vi "DestroyPublicEvents.vi"(8 "error in (no error)":errorcluster, 11 "SMO.Configurable":refnum<class "SMO.Configurable.lvclass">) -> (0 "error out":errorcluster, 3 "SMO.Configurable out":refnum<class "SMO.Configurable.lvclass">)   [LabVIEW 2013, in "SMO.Configurable.lvclass"]
uses:
  SMO.Configurable.lvclass
  src/SMO/SMO.lvclass
  SMO.Configurable.lvclass/SMO.Configurable.ctl
panel:
  # "For instructions on how to use the JKI State Machine Objects, examples and video tutorials, visit:\nhttp://jki.net/state-machine-objects/\n\nJKI State Machine Objects™\nhttp://jki.net/state-machine-objects/\nCopyright (C) 2005-2015, JKI <info@jki.net>\nALL RIGHTS RESERVED"
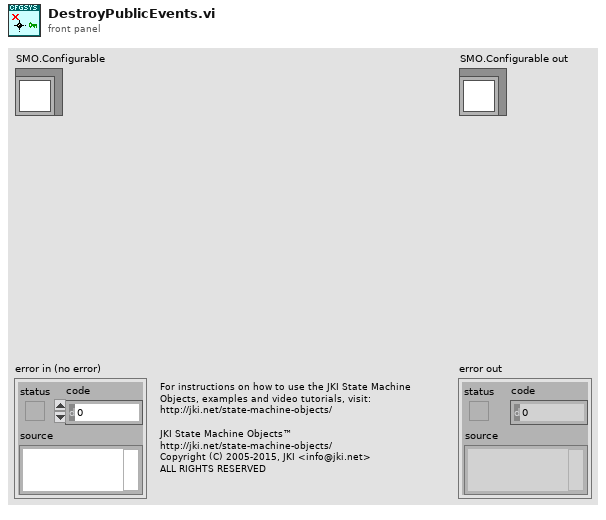
[diagram p1: front panel]
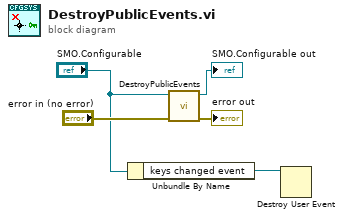
[diagram p0: block diagram]
diagram:
  n1 = Unbundle By Name("SMO.Configurable") -> ("keys changed event"=w1:refnum<user-event>)
  n2 = call-parent "DestroyPublicEvents.vi"("error in (no error)"="error in (no error)", "SMO"="SMO.Configurable") -> ("error out"=→"error out":errorcluster, "SMO out"=→"SMO.Configurable out":refnum<class "SMO.Configurable.lvclass">)  [unwired: 8 in]
  n3 = Destroy User Event(user event=w1) -> ()  [unwired: 1 in, 1 out]
